vi "citTemplate.ErrorEventPass.vi"(7 "instance":i32, 8 "error in (no error)":errorcluster, 10 "action of error":variant, 11 "event in":variant) -> (0 "error out":errorcluster)   [LabVIEW 2019, in "Tools.lvlib"]
uses:
  Tools.lvlib
  citTemplate.errData.ctl
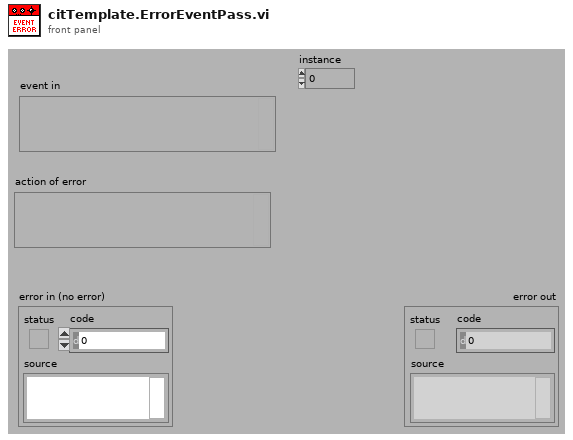
[diagram p1: front panel]
types:
  T1 = typedef "Tools.lvlib/citTemplate.errData.ctl" = cluster{"action":string, "error":errorcluster}
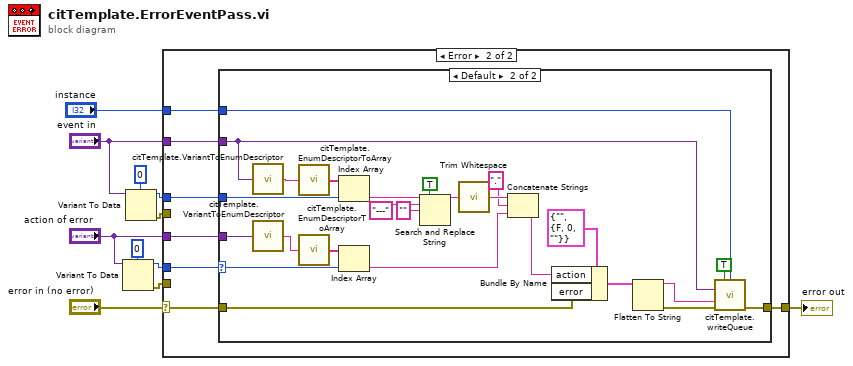
[diagram p0: block diagram]
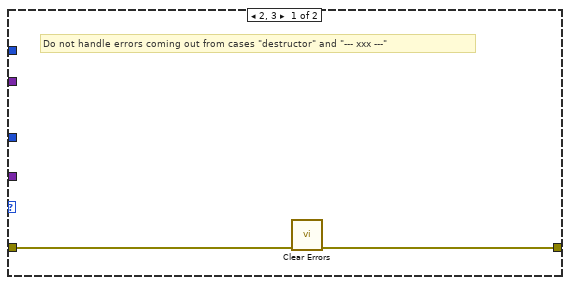
[diagram p3: hidden frame]
diagram:
  n1 = Variant To Data(type=u32 0 ("u32"), Variant="action of error") -> (data=w6:u32, error out=w7:errorcluster)  [unwired: 1 in]
  n2 = Variant To Data(type=u32 0 ("u32"), Variant="event in") -> (data=w2:u32, error out=w3:errorcluster)  [unwired: 1 in]
  n3 = case shown="Error" "error in (no error)" {
    selector: "error in (no error)" -> [w12 w15]
    tunnel: [w12 w19] -> w10
    tunnel: "event in" -> [_ w18]
    tunnel: "action of error" -> [_ w17]
    tunnel: w7 -> [_ _]
    tunnel: w6 -> [_ w13]
    tunnel: w3 -> [_ _]
    tunnel: w2 -> [_ w16]
    tunnel: "instance" -> [_ w14]
    frame No Error {
    }
    frame Error {
      n4 = case shown="Default" w13 {
        selector: w13 -> [_ w33]
        tunnel: [w20 w46] -> w19
        tunnel: w18 -> [_ w41]
        tunnel: w17 -> [_ w40]
        tunnel: w16 -> [_ w35]
        tunnel: w15 -> [w21 w25]
        tunnel: w14 -> [_ w34]
        frame 2, 3 {
          # "Do not handle errors coming out from cases \"destructor\" and \"--- xxx ---\""
          n5 = call <vilib>:"Clear Errors.vi"("error in (no error)"=w21) -> ("error out"=w20:errorcluster)  [unwired: 5 in, 1 out]
        }
        frame Default {
          n6 = call "citTemplate.VariantToEnumDescriptor.vi"("Variant enum data"=w41) -> ("enum type descriptor"=w36:string)  [unwired: 14 out]
          n7 = call "citTemplate.VariantToEnumDescriptor.vi"("Variant enum data"=w40) -> ("enum type descriptor"=w39:string)  [unwired: 14 out]
          n8 = call "citTemplate.EnumDescriptorToArray.vi"("enum type descriptor"=w36) -> ("array"=w37:string[])  [unwired: 14 out]
          n9 = call "citTemplate.EnumDescriptorToArray.vi"("enum type descriptor"=w39) -> ("array"=w38:string[])  [unwired: 14 out]
          n10 = Index Array(array=w37, index=w35) -> (element=w31:string)
          n11 = Index Array(array=w38, index=w33) -> (element=w23:string)
          n12 = Search and Replace String(replace all?=TRUE ("replace all? (F)"), input string=w31, search string="---" ("substring (\"\")"), replace string="" ("replace string (\"\")")) -> (result string=w30:string)  [unwired: 4 in, 3 out]
          n13 = call <vilib>:"Trim Whitespace.vi"("string"=w30) -> ("trimmed string"=w26:string)  [unwired: 1 in]
          n14 = Concatenate Strings(w26, "." ("string"), w23) -> (w24:string)
          n15 = Bundle By Name(cluster=T1 {"action"="", "error"={"status"=FALSE, "code"=0, "source"=""}} ("ErrData"), "action"=w24, "error"=w25) -> (w43:T1)
          n16 = Flatten To String(anything=w43) -> (data string=w44:string, error out=w45:errorcluster)  [unwired: 2 in, 2 out]
          n17 = call "citTemplate.writeQueue.vi"("High priority (F)"=TRUE, "instance (0)"=w34, "event in (if not connected:all statemachine with data event)"=w41, "data in"=w44, "error in (no error)"=w45) -> ("error out"=w46:errorcluster)  [unwired: 10 out]
        }
      }
    }
  }
  "error out" <- w10
